vi "Run Action_Do.vi"(8 "error in (no error)":errorcluster, 11 "Report":refnum<class "Report Action.lvclass">) -> (0 "error out":errorcluster, 1 "Success?":bool, 3 "Report Array":refnum<class "Report Data.lvclass">[](array[class]))   [LabVIEW 2020, in "ProjectBuilder.lvlib" / "Report Action.lvclass"]
uses:
  Report Action.lvclass
  Data/Report Data/Report Data.lvclass
  Action/Project Action/Project Action.lvclass
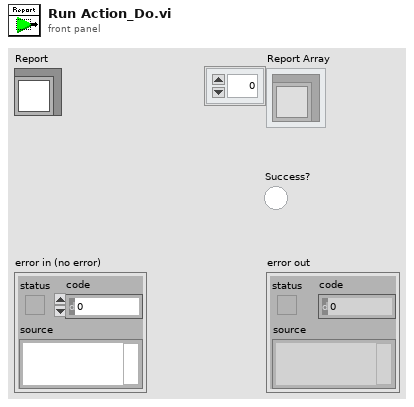
[diagram p1: front panel]
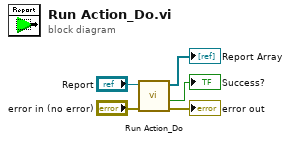
[diagram p0: block diagram]
diagram:
  n1 = call-parent "Run Action_Do.vi"("error in (no error)"="error in (no error)", "Project Action"="Report") -> ("error out"=→"error out":errorcluster, "Success?"=→"Success?":bool, "Report Array"=→"Report Array":refnum<class "Report Data.lvclass">[])  [unwired: 7 in]
